vi "Defer Top Level Updates.vi"(5 "error in (no error)":errorcluster, 6 "Defer Panel Updates (f)":bool) -> (1 "error out":errorcluster)   [LabVIEW 2013]
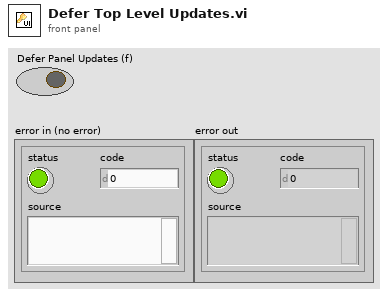
[diagram p1: front panel]
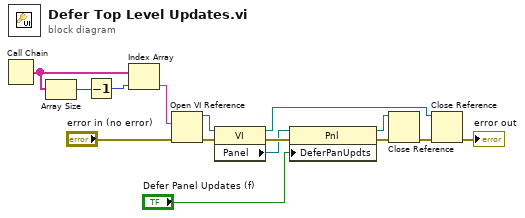
[diagram p0: block diagram]
diagram:
  n1 = Call Chain() -> (call chain=w9:string[])
  n2 = Array Size(array=w9) -> (size(s)=w7:i32)
  n3 = Decrement(x=w7) -> (x-1=w8:i32)
  n4 = Index Array(array=w9, index=w8) -> (element=w10:string)
  n5 = Open VI Reference(vi path=w10, error in (no error)="error in (no error)") -> (vi reference=w11:refnum<vi>, error out=w12:errorcluster)  [unwired: 4 in]
  n6 = property class="VI"(reference=w11, error in=w12) -> (reference out=w3:refnum<vi>, error out=w14:errorcluster, "Panel"=w13:refnum<vi>)
  n7 = property class="Pnl"(reference=w13, error in=w14, "DeferPanUpdts"="Defer Panel Updates (f)") -> (reference out=w6:refnum<vi>, error out=w4:errorcluster)
  n8 = Close Reference(reference=w6, error in (no error)=w4) -> (error out=w5:errorcluster)
  n9 = Close Reference(reference=w3, error in (no error)=w5) -> (error out=→"error out":errorcluster)
